vi "Configure Average.vi"(7 "Average On":bool, 8 "error in (no error)":errorcluster, 10 "Number of Averages":i32, 11 "VNA-ENA in":refnum<class "VNA-ENA.lvclass">) -> (0 "error out":errorcluster, 3 "VNA-ENA out":refnum<class "VNA-ENA.lvclass">)   [LabVIEW 2020, in "VNA-ENA.lvclass"]
doc: "Configures the average to use for the sweep"
uses:
  VNA-ENA.lvclass
  C:/Sandbox/Git_Sandbox/WiSpry Test Framework source code (LV20)/WiSpry Test Framework/Instruments/Instrument.lvclass
  Instrument.lvclass/Instrument.ctl
  Instrument.lvclass
  <instrlib>/Agilent ENA Series/Agilent ENA Series.lvlib
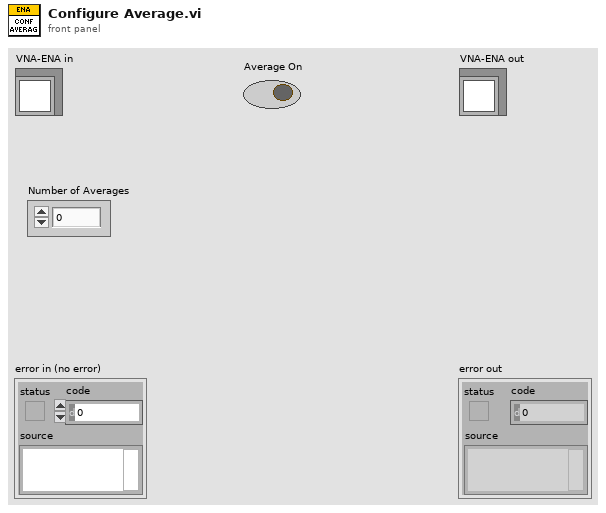
[diagram p1: front panel]
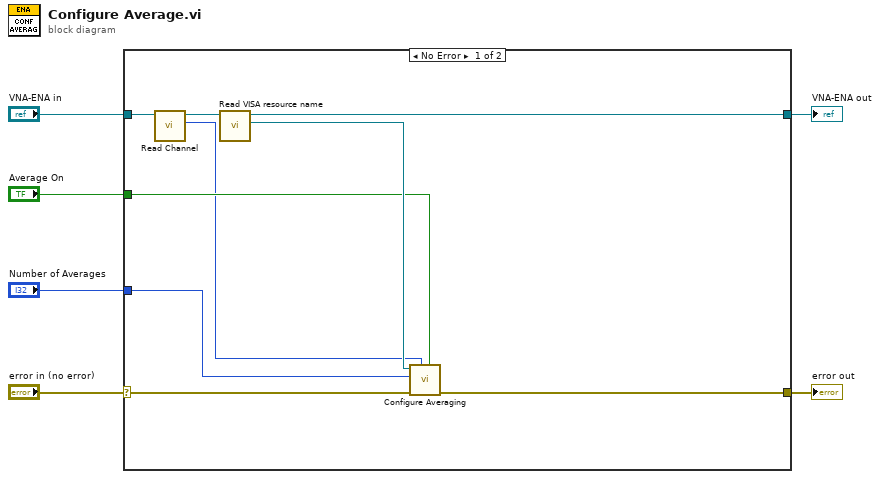
[diagram p0: block diagram]
diagram:
  n1 = case shown="No Error" "error in (no error)" {
    selector: "error in (no error)" -> [w14 w17]
    tunnel: [w13 w17] -> w5
    tunnel: [w15 w16] -> w4
    tunnel: "VNA-ENA in" -> [w8 w16]
    tunnel: "Number of Averages" -> [w11 _]
    tunnel: "Average On" -> [w10 _]
    frame No Error {
      n2 = call-dynamic "Read Channel.vi"("Vector Network Analyzer in"=w8) -> ("Channel"=w7:i32, "Vector Network Analyzer out"=w9:refnum<class "VNA-ENA.lvclass">)  [unwired: 9 in]
      n3 = call "Read VISA resource name.vi"("Instrument in"=w9) -> ("VISA resource name"=w12:refnum<visa-resource-name>, "Instrument out"=w15:refnum<class "VNA-ENA.lvclass">)  [unwired: 9 in]
      n4 = call <instrlib>:"Configure Averaging.vi"("Averaging State (F: Off)"=w10, "Channel (1)"=w7, "error in (no error)"=w14, "Factor (16)"=w11, "VISA resource name"=w12) -> ("error out"=w13:errorcluster)  [unwired: 5 in, 1 out]
    }
    frame Error {
    }
  }
  "error out" <- w5
  "VNA-ENA out" <- w4
